vi "Configure Speed.vi"(8 "error in (no error)":errorcluster, 10 "Speed (1500 us)":i32=1500, 11 "TI MDL BDC24 Simulator in":refnum<class "TI MDL BDC24 Simulator.lvclass">) -> (0 "error out":errorcluster, 3 "TI MDL BDC24 Simulator out":refnum<class "TI MDL BDC24 Simulator.lvclass">)   [LabVIEW 2012]
doc: "Configures the speed and direction."
uses:
  <vilib>/robotics/Simulator/Robot Factory/Motor/ODESimulator_Motor.lvclass
  <instrlib>/TI MDL BDC24/HAIOL/Simulator/TI MDL BDC24 Simulator.lvclass
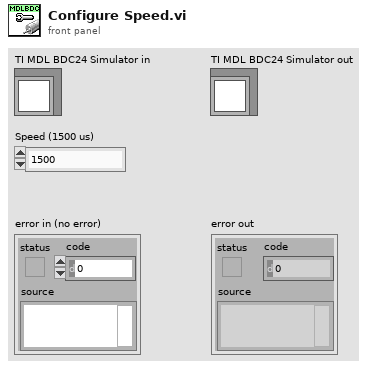
[diagram p1: front panel]
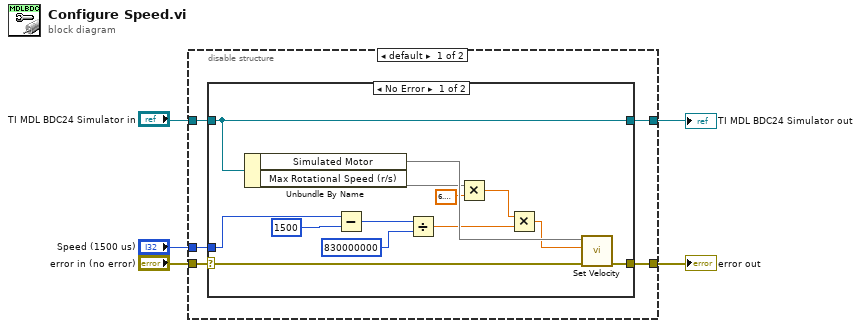
[diagram p0: block diagram]
diagram:
  n1 = disable-structure shown="default" {
    disable-tunnel: "error in (no error)" -> [w10 w26]
    disable-tunnel: "TI MDL BDC24 Simulator in" -> [w9 w27]
    disable-tunnel: [w8 w27] -> w1
    disable-tunnel: [w7 w26] -> w4
    disable-tunnel: "Speed (1500 us)" -> [w6 _]
    frame condition #0 (active) {
      n2 = case shown="No Error" w10 {
        selector: w10 -> [w22 w24]
        tunnel: w9 -> [w23 w25]
        tunnel: [w23 w25] -> w8
        tunnel: [w20 w24] -> w7
        tunnel: w6 -> [w19 _]
        frame No Error {
          n3 = Unbundle By Name(w23) -> ("Simulated Motor"=w21, "Max Rotational Speed (r/s)"=w14)
          n4 = Subtract(x=w19, y=1500) -> (x-y=w17:i32)
          n5 = Divide(x=w17, y=830000000) -> (x/y=w15:dbl)
          n6 = Multiply(x=w14, y=6.283185307179586) -> (x*y=w12:dbl)
          n7 = Multiply(x=w12, y=w15) -> (x*y=w11:dbl)
          n8 = call-dynamic "Set Velocity.vi"("error in (no error)"=w22, "CCW Velocity (0.0 rad/s)"=w11, "Motor in"=w21) -> ("error out"=w20:errorcluster)  [unwired: 7 in, 1 out]
        }
        frame Error {
        }
      }
    }
    frame condition #1 {
    }
  }
  "error out" <- w4
  "TI MDL BDC24 Simulator out" <- w1
